vi "Project Items.vi"(8 "error in (no error)":errorcluster, 9 "Exclude":T1, 11 "Project in":refnum<vi>) -> (0 "error out":errorcluster, 1 "Symbol Array":T3(array[cluster]), 2 "Items":T2(array[cluster]), 3 "Project out":refnum<vi>)   [LabVIEW 2018]
panel:
  in  "Tree":string(tree)
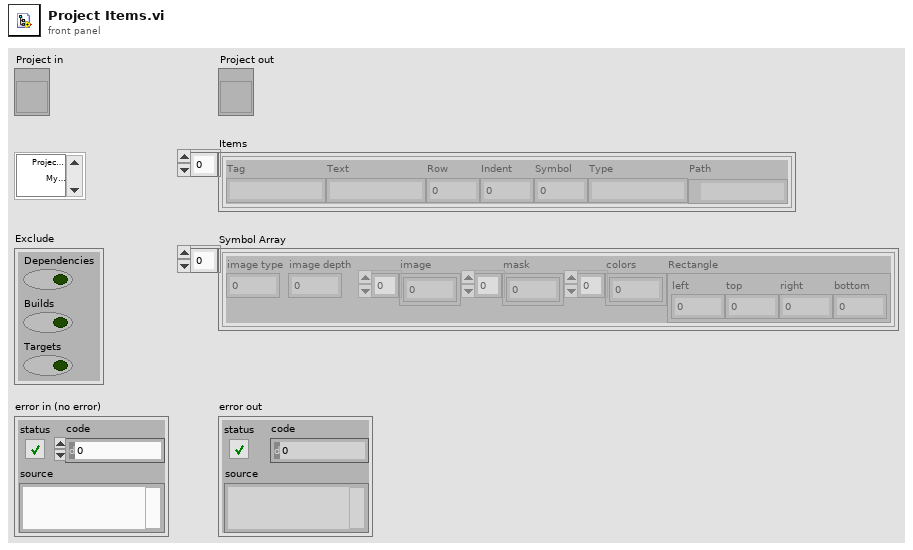
[diagram p1: front panel]
types:
  T1 = cluster{"Dependencies":bool, "Builds":bool, "Targets":bool}
  T2 = cluster{"Tag":string, "Text":string, "Row":i32, "Indent":i32, "Symbol":i32, "Type":string, "Path":path}[]
  T3 = cluster{"image type":i32, "image depth":i32, "image":u8[], "mask":u8[], "colors":u32[], "Rectangle":cluster{"left":i16, "top":i16, "right":i16, "bottom":i16}}[]
  T4 = cluster{"Tag":string, "Text":string, "Row":i32, "Indent":i32, "Symbol":i32, "Type":string, "Path":path}
  T5 = cluster{"image type":i32, "image depth":i32, "image":u8[], "mask":u8[], "colors":u32[], "Rectangle":cluster{"left":i16, "top":i16, "right":i16, "bottom":i16}}
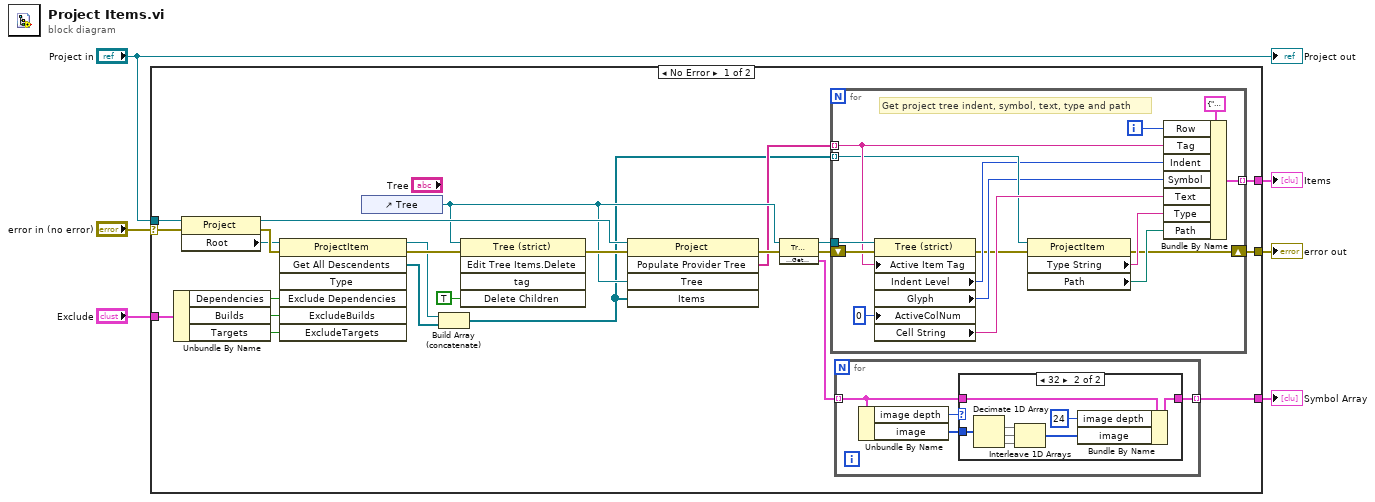
[diagram p0: block diagram]
diagram:
  n1 = case shown="No Error" "error in (no error)" {
    selector: "error in (no error)" -> [w20 w59]
    tunnel: [w12 _] -> w6
    tunnel: [w22 _] -> w5
    tunnel: [w19 w59] -> w3
    tunnel: "Project in" -> [w18 _]
    tunnel: "Exclude" -> [w17 _]
    frame No Error {
      n2 = Unbundle By Name(w17) -> ("Dependencies"=w16:bool, "Builds"=w15:bool, "Targets"=w14:bool)
      n3 = property class="Project"(reference=w18, error in=w20) -> (reference out=w29:refnum<vi>, error out=w30:errorcluster, "Root"=w27:refnum<vi>)
      n4 = invoke class="ProjectItem" method="Get All Descendents"(reference=w27, error in=w30, "Exclude Dependencies"=w16, "ExcludeBuilds"=w15, "ExcludeTargets"=w14) -> (reference out=w11:refnum<vi>, error out=w28:errorcluster, "All Descendents"=w26:refnum<vi>[])  [unwired: 2 in, 4 out]
      n5 = control-ref of="Tree"() -> (w24:refnum<vi>)
      n6 = Build Array (concatenate)(w11, w26) -> (w8:refnum<vi>[])
      n7 = invoke class="Tree (strict)" method="Edit Tree Items.Delete"(reference=w24, error in=w28, "Delete Children"=TRUE ("Delete Children?")) -> (error out=w25:errorcluster)  [unwired: 2 in, 4 out]
      n8 = invoke class="Project" method="Populate Provider Tree"(reference=w29, error in=w25, "Tree"=w24, "Items"=w8) -> (error out=w21:errorcluster, "Populate Provider Tree"=w9:string[])  [unwired: 1 in, 3 out]
      n9 = invoke class="Tree (strict)" method="Custom Item Symbols.Get Symbol Array"(reference=w24, error in=w21) -> (reference out=w7:refnum<vi>, error out=w10:errorcluster, "Custom Glyphs:Get Glyph Array"=w13:T3)  [unwired: 1 in]
      n10 = for {
        tunnel: w7 -> [w45]
        tunnel: w9 -> [w43] mode=indexing
        tunnel: [w41] -> w22 mode=indexing
        shift-right: [w31] -> w19
        shift-left: w10 -> [w44]
        tunnel: w8 -> [w38] mode=indexing
        i -> [w35]
        # "Get project tree indent, symbol, text, type and path"
        n11 = property class="Tree (strict)"(reference=w45, error in=w44, "Active Item Tag"=w43, "ActiveColNum"=0 ("Active Cell:Active Column Number")) -> (error out=w32:errorcluster, "Indent Level"=w34:i32, "Glyph"=w33:i32, "Cell String"=w40:string)  [unwired: 1 out]
        n12 = property class="ProjectItem"(reference=w38, error in=w32) -> (error out=w31:errorcluster, "Type String"=w37:string, "Path"=w36:path)  [unwired: 1 out]
        n13 = Bundle By Name(cluster=T4 {"Tag"="", "Text"="", "Row"=0, "Indent"=0, "Symbol"=0, "Type"="", "Path"=path ""} ("Item"), "Row"=w35, "Tag"=w43, "Indent"=w34, "Symbol"=w33, "Text"=w40, "Type"=w37, "Path"=w36) -> (w41:T4)
      }
      n14 = for {
        tunnel: w13 -> [w46] mode=indexing
        tunnel: [w47] -> w12 mode=indexing
        n15 = Unbundle By Name(w46) -> ("image depth"=w49:i32, "image"=w48:u8[])
        n16 = case shown="32" w49 {
          tunnel: w48 -> [_ w56]
          tunnel: [w50 w57] -> w47
          tunnel: w46 -> [w50 w58]
          frame Default {
          }
          frame 32 {
            n17 = Decimate 1D Array(w56) -> (w54:u8[], w53:u8[], w52:u8[])  [unwired: 1 out]
            n18 = Interleave 1D Arrays(w54, w53, w52) -> (w51:u8[])
            n19 = Bundle By Name(cluster=w58, "image depth"=24, "image"=w51) -> (w57:T5)
          }
        }
      }
    }
    frame Error {
    }
  }
  "Symbol Array" <- w6
  "Items" <- w5
  "error out" <- w3
  "Project out" <- "Project in"
